vi "Present.vi"(6 "Reverse Rows (T)":bool=TRUE, 11 "Pixel Data in":u32[][](array[numeric])) -> (3 "2D Picture":picture)   [LabVIEW 2020, in "Raster.lvlib"]
uses:
  Raster.lvlib
  <vilib>/Utility/High Resolution Relative Seconds.vi
  <vilib>/picture/picture.llb/Draw True-Color Pixmap.vi
  Utility/Utility.lvlib
panel:
  out "Present Time [s]":dbl format="%.1p"
  # "(0,0)"
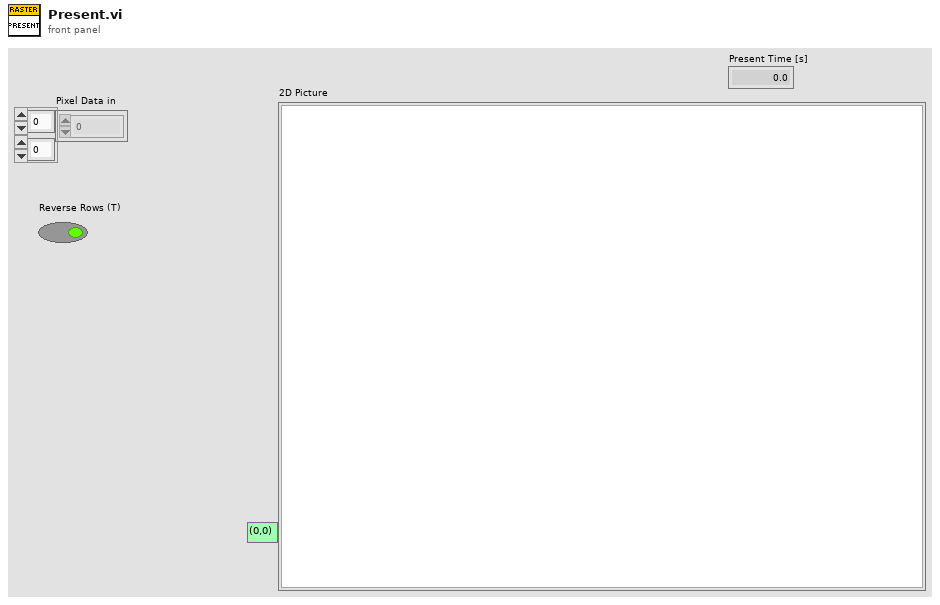
[diagram p1: front panel]
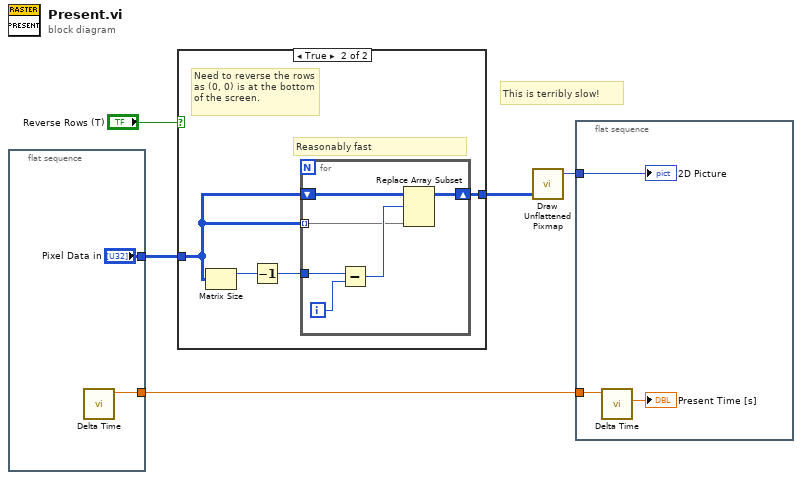
[diagram p0: block diagram]
diagram:
  # "This is terribly slow!"
  n1 = flat-sequence {
    tunnel: ["Pixel Data in"] -> w4
    tunnel: [w6] -> w1
    frame #0 {
      n2 = call "Delta Time.vi"() -> ("Relative Seconds Out"=w6:dbl)  [unwired: 10 in, 1 out]
    }
  }
  n3 = case shown="True" "Reverse Rows (T)" {
    tunnel: w4 -> [w8 w12]
    tunnel: [w8 w9] -> w2
    frame False {
    }
    frame True {
      # "Need to reverse the rows as (0, 0) is at the bottom of the screen."
      # "Reasonably fast"
      n4 = Matrix Size(0:w12) -> (1:w11:i32)  [unwired: 1 out]
      n5 = Decrement(x=w11) -> (x-1=w10:i32)
      n6 = for {
        tunnel: w12 -> [w14] mode=indexing
        shift-right: [w13] -> w9
        shift-left: w12 -> [w18]
        tunnel: w10 -> [w17]
        i -> [w16]
        n7 = Subtract(x=w17, y=w16) -> (x-y=w15:i32)
        n8 = Replace Array Subset(array=w18, new element=w14, index (row)=w15) -> (w13:u32[][])  [unwired: 1 in]
      }
    }
  }
  n9 = call-poly <vilib>:"Draw Unflattened Pixmap.vi"("data (RGB format)"=w2) -> ("new picture"=w5:picture)  [unwired: 8 in]
  n10 = flat-sequence {
    tunnel: w5 -> [w21]
    tunnel: w1 -> [w20]
    frame #0 {
      n11 = call "Delta Time.vi"("Relative Seconds In"=w20) -> ("Delta Seconds"=→"Present Time [s]":dbl)  [unwired: 9 in, 1 out]
      "2D Picture" <- w21
    }
  }
